vi "Seno Subvi.vi"(10 "Fase Inicial":fxp<+,27,1>, 11 "Phase Inc Corriente":fxp<+,27,0>=0.00020000338554382324) -> (3 "sin(x)":fxp<+/-,16,2>)   [LabVIEW 2020]
uses:
  <vilib>/rvi/FXPMathLib/FxpSinAndCos/subVIs/nifxpmath_SinAndCos_SimConfig.ctl
  <vilib>/rvi/FXPMathLib/FxpSinAndCos/simVIs/DllFxpSinAndCosTemp_sub.vi
  <vilib>/rvi/FXPMathLib/FxpAdd/XNode/nifxpmath_Add.xnode
  <vilib>/rvi/FXPMathLib/FxpSinAndCos/XNode/nifxpmath_SinAndCos.xnode
  <vilib>/rvi/FXPMathLib/sim/FxpSim.dll
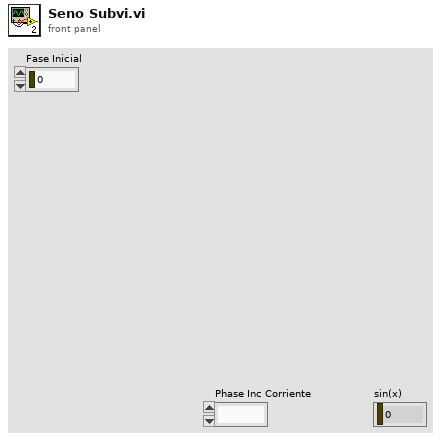
[diagram p1: front panel]
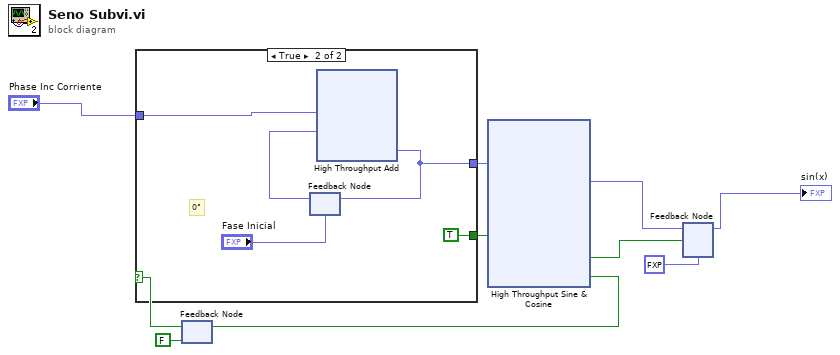
[diagram p0: block diagram]
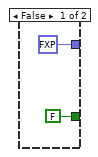
[diagram p2: hidden frame]
diagram:
  n1 = feedback #1(FALSE ("ready for input")) -> (w6:bool)
  n2 = case shown="True" w6 {
    tunnel: "Phase Inc Corriente" -> [_ w17]
    tunnel: [fxp<+/-,16,1> 0.0 ("x+y") w14] -> w8
    tunnel: [FALSE TRUE] -> w7
    frame False {
    }
    frame True {
      # "0°"
      n3 = feedback #2("Fase Inicial") -> (w15:fxp<+,27,1>)
      n4 = xnode ("High Throughput Add")("x"=w17, "y"=w15) -> ("x+y"=w14:fxp<+,27,1>)
      n5 = feedback-in #2(w14) -> ()
    }
  }
  n6 = xnode "High Throughput Sine & Cosine"("x (pi)"=w8, "input valid"=w7) -> ("sin(x)"=w3:fxp<+/-,16,2>, "output valid"=w4:bool, "ready for input"=w9:bool)  [unwired: 1 in, 1 out]
  n7 = feedback-in #1(w9) -> ()
  n8 = feedback-in #3(w3, w4) -> ()
  n9 = feedback #3(fxp<+/-,16,2> 0.0 ("sin(x)")) -> (→"sin(x)":fxp<+/-,16,2>)
